vi "SendAxisMoveCmd.vi"(8 "Instant? (T)":bool=TRUE, 9 "Speed":sgl, 10 "axis":T1, 11 "Position":sgl) -> (3 "Limited pos":dbl)   [LabVIEW 2011]
uses:
  MotorAxisEnum.ctl
  Typedefs/CmdEnum_MotorIn.ctl
  MotorCmd_SetPosition.ctl
  GlobalVariables.vi
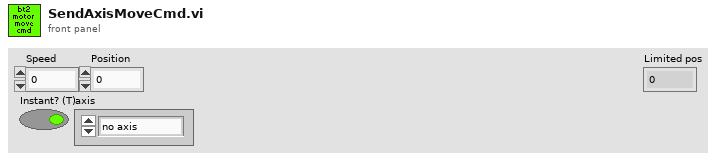
[diagram p1: front panel]
types:
  T1 = typedef "MotorAxisEnum.ctl" = enum16{"no axis", "magrot", "magpos", "px", "py", "pz", "camx", "camy"}
  T2 = typedef "MotorCmd_SetPosition.ctl" = cluster{"Position":dbl, "Speed":sgl, "Instant?":bool, "Motor Axis":T1}
  T3 = typedef "CmdEnum_MotorIn.ctl" = enum32{"Init", "Close", "SetPosition", "UpdatePositions", "MoveToLimit"}
  T4 = typedef "MotorConfigType.ctl" = cluster{"Offset":T5, "Maximum pos":T5, "Min limited?":T7, "Max limited?":T7, "Has velocity support":T7, "Default velocity":T5}
  T5 = typedef "MotorPosType.ctl" = cluster{"Magnet Z":dbl, "Magnet rotation":dbl, "Camera":T6, "Piezo XY":T6, "Piezo Z":dbl}
  T6 = typedef "XYf.ctl" = cluster{"X":sgl, "Y":sgl}
  T7 = typedef "MotorPosFlagsType.ctl" = cluster{"Magnet Z":bool, "Magnet rotation":bool, "Camera":cluster{"X":bool, "Y":bool}, "Piezo XY":cluster{"X":bool, "Y":bool}, "Piezo Z":bool}
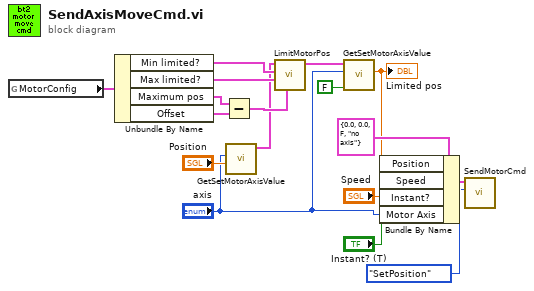
[diagram p0: block diagram]
diagram:
  n1 = global read "GlobalVariables.vi" "MotorConfig"() -> (w13:T4)
  n2 = Unbundle By Name(w13) -> ("Min limited?"=w16:T7, "Max limited?"=w15:T7, "Maximum pos"=w12:T5, "Offset"=w11:T5)
  n3 = Subtract(x=w12, y=w11) -> (x-y=w10:T5)
  n4 = call "GetSetMotorAxisValue.vi"("pos"="Position", "axis"="axis") -> ("Motorpos out"=w8:T5)  [unwired: 8 in, 1 out]
  n5 = call "LimitMotorPos.vi"("Maximum pos"=w10, "max limit"=w15, "Min limit"=w16, "Position in"=w8) -> ("Position out"=w7:T5)  [unwired: 7 in]
  n6 = call "GetSetMotorAxisValue.vi"("set? (T)"=FALSE, "axis"="axis", "Motorpos in"=w7) -> ("pos (out)"=w5:dbl)  [unwired: 7 in, 1 out]
  "Limited pos" <- w5
  n7 = Bundle By Name(cluster=T2 {"Position"=0.0, "Speed"=0.0, "Instant?"=FALSE, "Motor Axis"=enum."no axis"} ("SetMotorPosCmdData"), "Position"=w5, "Speed"="Speed", "Instant?"="Instant? (T)", "Motor Axis"="axis") -> (w17:T2)
  n8 = call "SendMotorCmd.vi"("Command Type"=CmdEnum_MotorIn."SetPosition", "Command Data"=w17) -> ()  [unwired: 10 in]
